vi "Main.vi"() -> ()   [LabVIEW 2014]
uses:
  <vilib>/Utility/config.llb/Read Key (Path).vi
  <vilib>/Utility/config.llb/NI_LVConfig.lvlib
panel:
  in  "stop":bool
  out "Spinny Lights":T1
  in  "Month":string="08"
  in  "Browse Button":bool
  in  "Base Save Path":path
  out "All Messages":T2(array[cluster])
  in  "Save Button":bool
  out "Report":string
  in  "Day":string="01"
  in  "Report":bool
  out "Error Codes":errorcluster
  in  "Expected Size":i32=343
  in  "IMEI":string="300234010864450"
  in  "stop":bool
  in  "Starting Path":string="/pub/outgoing/iridium/"
  in  "FTP Server":string="tidepool.nos.noaa.gov"
  # "Report Statistics"
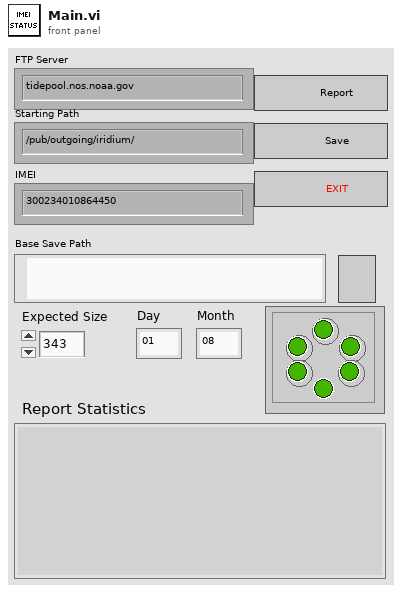
[diagram p1: front panel]
types:
  T1 = cluster{"1":bool, "2":bool, "3":bool, "4":bool, "5":bool, "6":bool}
  T2 = cluster{"name":string, "size":i32, "link name":string}[]
  T3 = typedef "NI_LVConfig.lvlib/Config Data RefNum.ctl" = refnum<k1>
  T4 = typedef "NI_FTP.lvlib/FTP File Info.ctl" = cluster{"type":enum16{"unknown", "file", "dir", "link"}, "permissions":string, "owner":string, "group":string, "size":i32, "date":string, "name":string, "link name":string}
  T5 = cluster{"String":string, "appended path":path, "binary":bool}[]
  T6 = cluster{"[0]":bool, "[1]":bool, "[2]":bool, "[3]":bool, "[4]":bool, "[5]":bool}
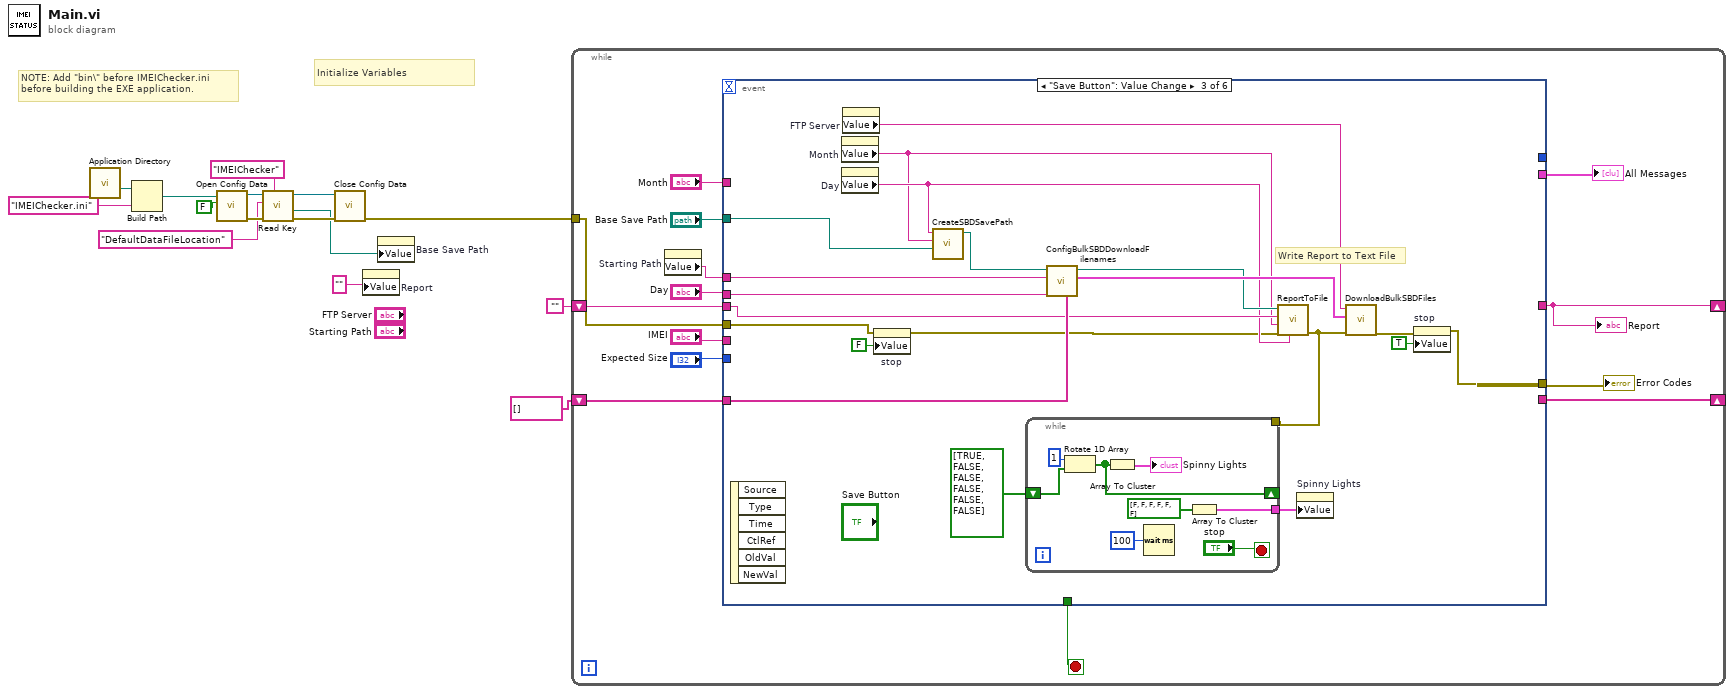
[diagram p0: block diagram]
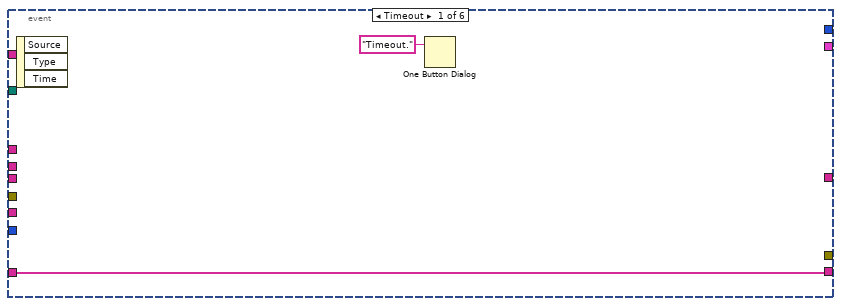
[diagram p2: hidden frame]
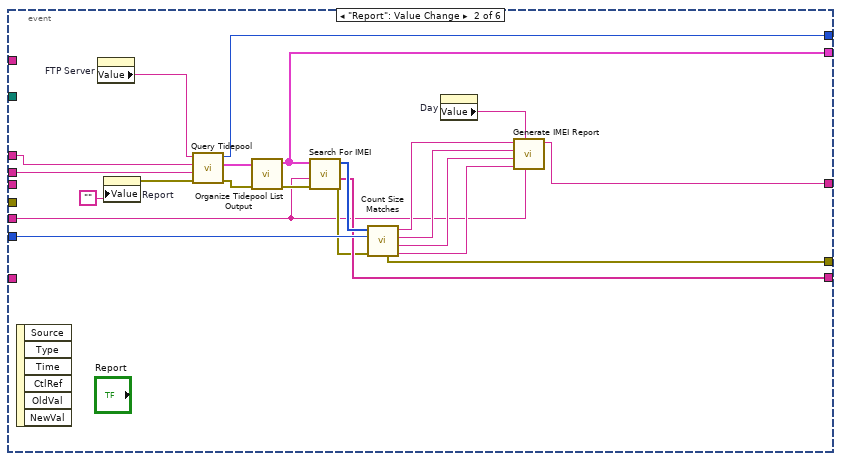
[diagram p3: hidden frame]
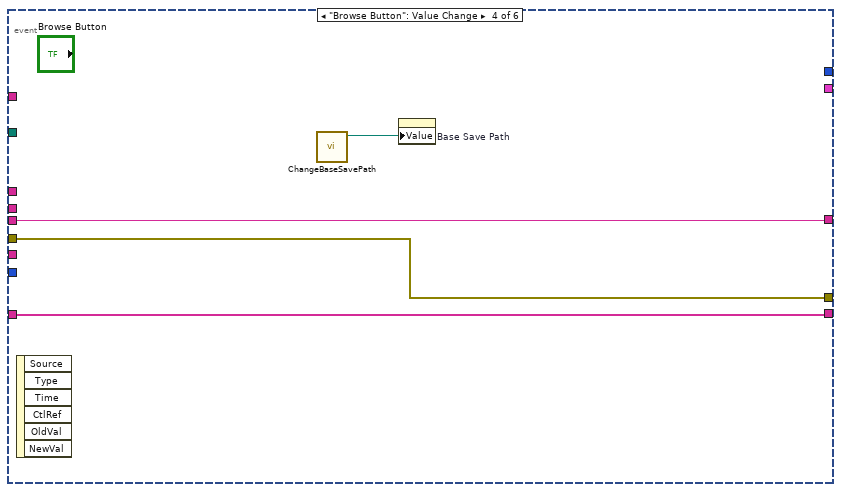
[diagram p4: hidden frame]
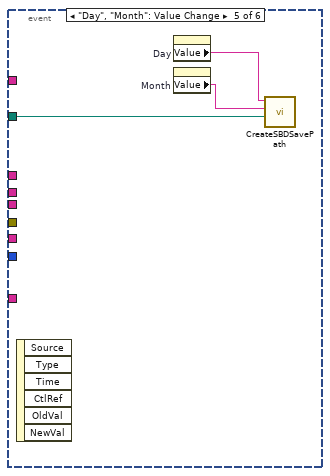
[diagram p5: hidden frame]
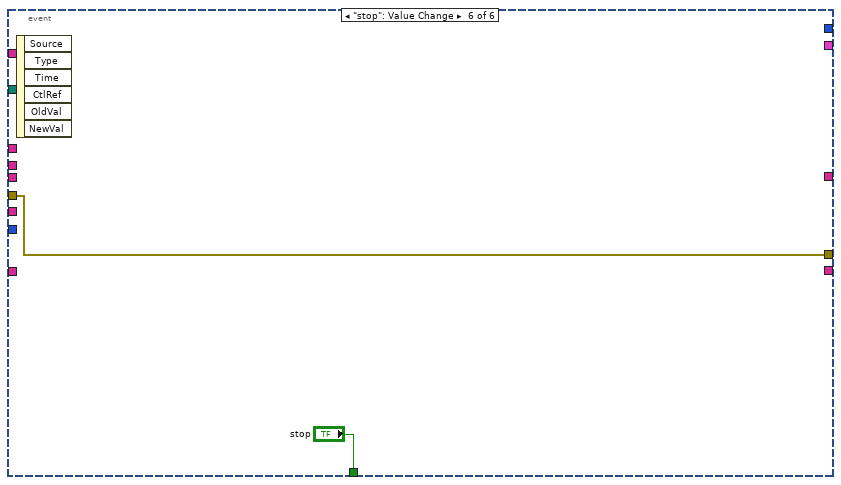
[diagram p6: hidden frame]
diagram:
  # "NOTE: Add \"bin\\\" before IMEIChecker.ini\nbefore building the EXE application."
  # "Initialize Variables"
  n1 = call <vilib>:"Application Directory.vi"() -> ("Application Directory"=w10:path)
  n2 = Build Path(base path=w10, name or relative path="IMEIChecker.ini") -> (appended path=w12:path)
  n3 = call <vilib>:"Open Config Data.vi"("create file if necessary (T)"=FALSE, "configuration file path"=w12) -> ("error out"=w8:errorcluster, "refnum"=w7:T3)  [unwired: 7 in, 1 out]
  n4 = call-poly <vilib>:"Read Key.vi"("section"="IMEIChecker", "error in (no error)"=w8, "key"="DefaultDataFileLocation", "refnum"=w7) -> ("error out"=w3:errorcluster, "value"=w2:path, "refnum out"=w4:T3)  [unwired: 4 in, 1 out]
  n5 = call <vilib>:"Close Config Data.vi"("error in (no error)"=w3, "refnum"=w4) -> ("error out"=w1:errorcluster)  [unwired: 8 in, 1 out]
  n6 = property on="Report" class="Str"("Value"="" ("Report")) -> ()  [unwired: 2 in, 2 out]
  n7 = property on="Base Save Path" class="Path"("Value"=w2) -> ()  [unwired: 2 in, 2 out]
  n8 = while {
    shift-right: [w26] -> _
    shift-left: "" -> [w25]
    shift-right: [w24] -> _
    shift-left: string[] [] ("Filenames") -> [w23]
    tunnel: w1 -> [w16]
    stop <- w29 stop-if-true
    n9 = property on="Starting Path" class="Str"() -> ("Value"=w22:string)  [unwired: 2 in, 2 out]
    n10 = event shown="[2] \"Save Button\": Value Change" {
      selector: _ -> [_ _ _ _ _ _]
      dyn-events: _ -> [_ _ _ _ _ _]
      timeout: _ -> [_ _ _ _ _ _]
      tunnel: [_ _ _ _ _ "stop"] -> w29
      tunnel: "IMEI" -> [_ w37 _ _ _ _]
      tunnel: "Expected Size" -> [_ w43 _ _ _ _]
      tunnel: [_ w53 _ _ _ _] -> _
      tunnel: [_ w52 _ _ _ _] -> w28
      tunnel: [_ w35 w60 w82 _ w89] -> w27
      tunnel: "Day" -> [_ w45 w72 _ _ _]
      tunnel: [_ w44 _ w85 _ _] -> w26
      tunnel: w25 -> [_ _ w67 w85 _ _]
      tunnel: "Base Save Path" -> [_ _ w63 _ w86 _]
      tunnel: [w30 w40 _ w84 _ _] -> w24
      tunnel: w23 -> [w30 _ w73 w84 _ _]
      tunnel: w22 -> [_ w32 w69 _ _ _]
      tunnel: "Month" -> [_ _ _ _ _ _]
      tunnel: w16 -> [_ _ w55 w82 _ w89]
      event Timeout {
        n11 = event-data() -> ()  [unwired: 1 in, 3 out]
        n12 = One Button Dialog(message="Timeout.") -> ()  [unwired: 1 in, 1 out]
      }
      event "Report": Value Change {
        n13 = event-data() -> ()  [unwired: 1 in, 6 out]
        n14 = property on="FTP Server" class="Str"() -> ("Value"=w42:string)  [unwired: 2 in, 2 out]
        n15 = property on="Report" class="Str"("Value"="") -> (error out=w36:errorcluster)  [unwired: 2 in, 1 out]
        n16 = call "Query Tidepool.vi"("error in (no error)"=w36, "Day"=w45, "Starting Path"=w32, "FTP Server"=w42) -> ("error out"=w41:errorcluster, "dir list"=w51:T4[], "Total SBD Files In Dir"=w53:i32)  [unwired: 5 in]
        n17 = call "Organize Tidepool List Output.vi"("error in"=w41, "dir list"=w51) -> ("error in 2"=w39:errorcluster, "Array"=w52:T2)  [unwired: 8 in]
        n18 = call "Search For IMEI.vi"("error in"=w39, "IMEI"=w37, "Array"=w52) -> ("error out"=w38:errorcluster, "Filenames"=w40:string[], "Sizes"=w50:i32[])  [unwired: 6 in]
        n19 = call "Count Size Matches.vi"("error in"=w38, "Expected Size in"=w43, "Sizes"=w50) -> ("% of Daily Expected Good"=w46:string, "% Good"=w47:string, "Daily SBD Messages (IMEI Match)"=w48:string, "Missed Tx (IMEI Match)"=w49:string, "error out"=w35:errorcluster)  [unwired: 4 in]
        n20 = property on="Day" class="Str"() -> ("Value"=w33:string)  [unwired: 2 in, 2 out]
        n21 = call "Generate IMEI Report.vi"("IMEI"=w37, "Day"=w33, "Daily Expected Tx % (IMEI Match):"=w46, "% Good Tx. (IMEI Match)"=w47, "Daily Tx (IMEI Match)"=w48, "Daily Missed Tx (IMEI Match)"=w49) -> ("Report"=w44:string)  [unwired: 5 in]
      }
      event "Save Button": Value Change {
        # "Write Report to Text File"
        n22 = event-data() -> ()  [unwired: 1 in, 6 out]
        n23 = property on="Month" class="Str"() -> ("Value"=w64:string)  [unwired: 2 in, 2 out]
        n24 = property on="Day" class="Str"() -> ("Value"=w65:string)  [unwired: 2 in, 2 out]
        n25 = property on="FTP Server" class="Str"() -> ("Value"=w71:string)  [unwired: 2 in, 2 out]
        n26 = property on="stop" class="Bool (strict)"(error in=w55, "Value"=FALSE) -> (error out=w54:errorcluster)  [unwired: 1 in, 1 out]
        n27 = call "CreateSBDSavePath.vi"("Base Save Path"=w63, "Month"=w64, "Day"=w65) -> ("File Path Control"=w66:path)  [unwired: 8 in]
        n28 = call "ConfigBulkSBDDownloadFilenames.vi"("Filenames"=w73, "Day"=w72, "Month"=w69, "Save Path"=w66) -> ("Array"=w70:T5, "dup path"=w68:path)  [unwired: 6 in]
        n29 = call "ReportToFile.vi"("Day"=w65, "error in"=w54, "Month"=w64, "Report"=w67, "dup path"=w68) -> ("error out"=w57:errorcluster)  [unwired: 6 in]
        n30 = while {
          shift-right: [w78] -> _
          shift-left: bool[] [TRUE, FALSE, FALSE, FALSE, FALSE, FALSE] -> [w79]
          tunnel: [w75] -> w61
          tunnel: w57 -> [_]
          stop <- "stop" stop-if-true
          n31 = Rotate 1D Array(1:w79, 2:1 ("n")) -> (0:w78:bool[])
          n32 = Array To Cluster(array=w78) -> (cluster=→"Spinny Lights":T6)
          n33 = Wait (ms)(milliseconds to wait=u32 100) -> ()  [unwired: 1 out]
          n34 = Array To Cluster(array=bool[] [FALSE, FALSE, FALSE, FALSE, FALSE, FALSE]) -> (cluster=w75:T6)
        }
        n35 = property on="Spinny Lights" class="Clust (strict)"("Value"=w61) -> ()  [unwired: 2 in, 2 out]
        n36 = call "DownloadBulkSBDFiles.vi"("error in (no error)"=w57, "Array"=w70, "Value"=w71) -> ("error out"=w58:errorcluster)  [unwired: 8 in]
        n37 = property on="stop" class="Bool (strict)"(error in=w58, "Value"=TRUE) -> (error out=w60:errorcluster)  [unwired: 1 in, 1 out]
      }
      event "Browse Button": Value Change {
        n38 = event-data() -> ()  [unwired: 1 in, 6 out]
        n39 = call "ChangeBaseSavePath.vi"() -> ("selected path"=w83:path)  [unwired: 11 in]
        n40 = property on="Base Save Path" class="Path"("Value"=w83) -> ()  [unwired: 2 in, 2 out]
      }
      event "Day", "Month": Value Change {
        n41 = event-data() -> ()  [unwired: 1 in, 6 out]
        n42 = property on="Day" class="Str"() -> ("Value"=w88:string)  [unwired: 2 in, 2 out]
        n43 = property on="Month" class="Str"() -> ("Value"=w87:string)  [unwired: 2 in, 2 out]
        n44 = call "CreateSBDSavePath.vi"("Base Save Path"=w86, "Month"=w87, "Day"=w88) -> ()  [unwired: 8 in, 1 out]
      }
      event "stop": Value Change {
        n45 = event-data() -> ()  [unwired: 1 in, 6 out]
      }
    }
    "Error Codes" <- w27
    "Report" <- w26
    "All Messages" <- w28
  }
